vi "Curve Generator (SubVI).vi"(4 "Number of Samples":i32, 6 "Total Length (ms)":dbl, 7 "Start Amplitude (mA)":dbl, 9 "Post-ramp\nRadius (ms/mA)":dbl, 10 "Pre-ramp\nRadius (ms/mA)":dbl, 11 "End Amplitude (mA)":dbl) -> (1 "Charge (mC)":dbl, 2 "dt":dbl, 3 "S-Curve":dbl[](array[numeric]))   [LabVIEW 2020]
uses:
  <vilib>/Analysis/1siggen.llb/Ramp Pattern by Samples.vi
  <vilib>/Analysis/NI_AALBase.lvlib
panel:
  out "output variable":dbl
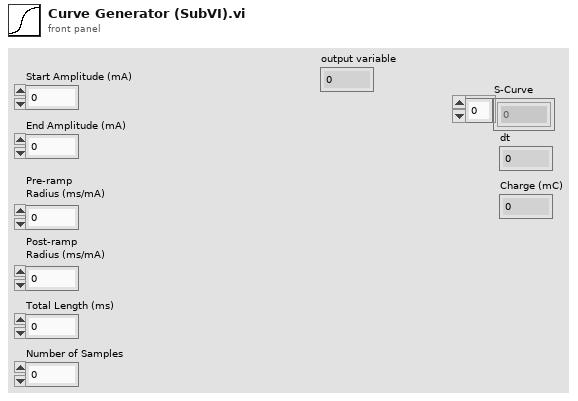
[diagram p1: front panel]
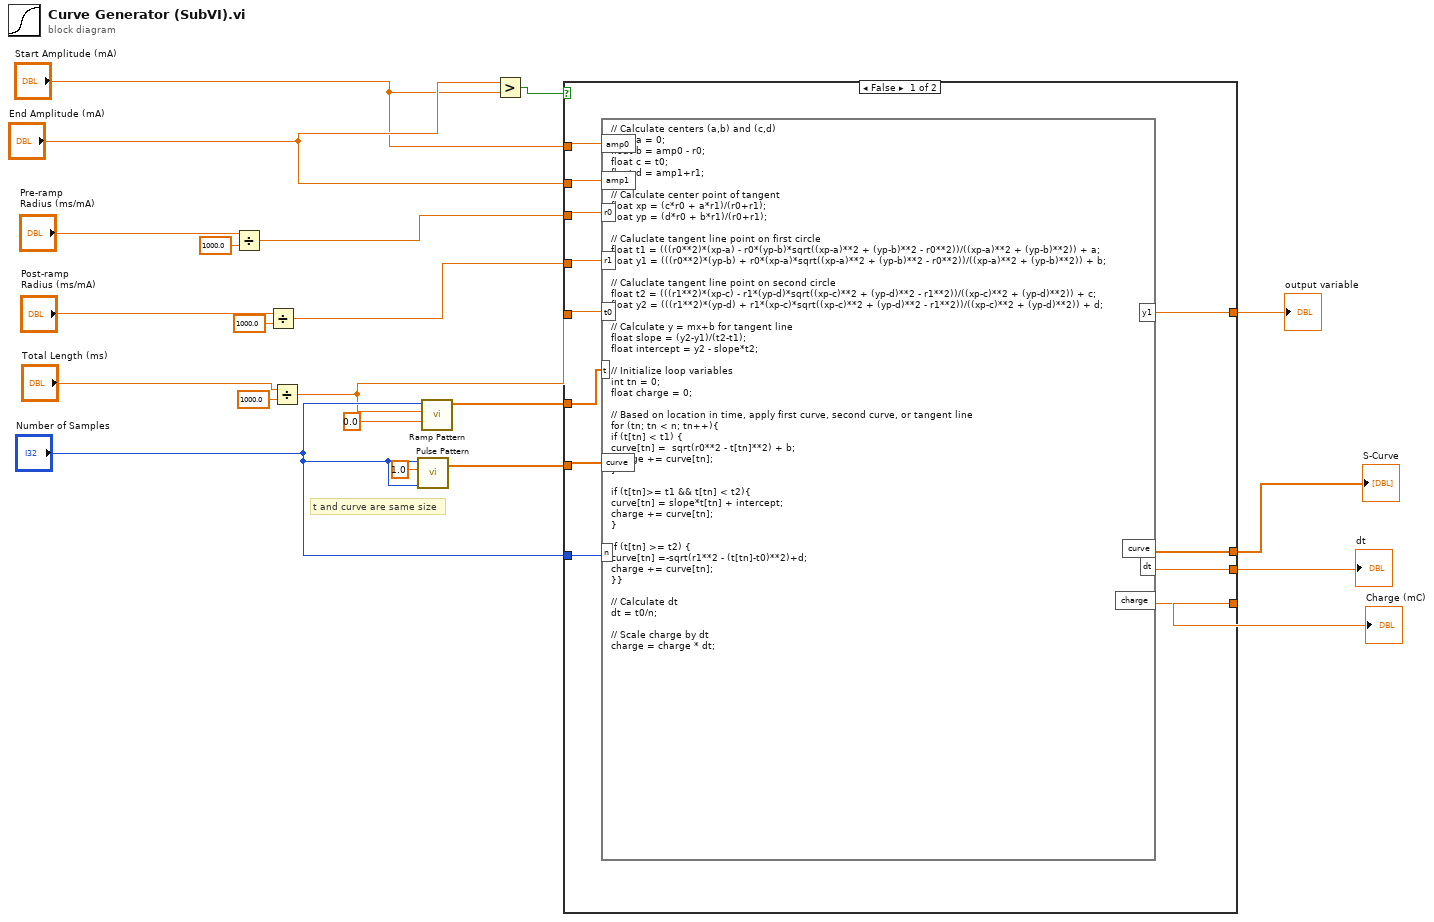
[diagram p0: block diagram]
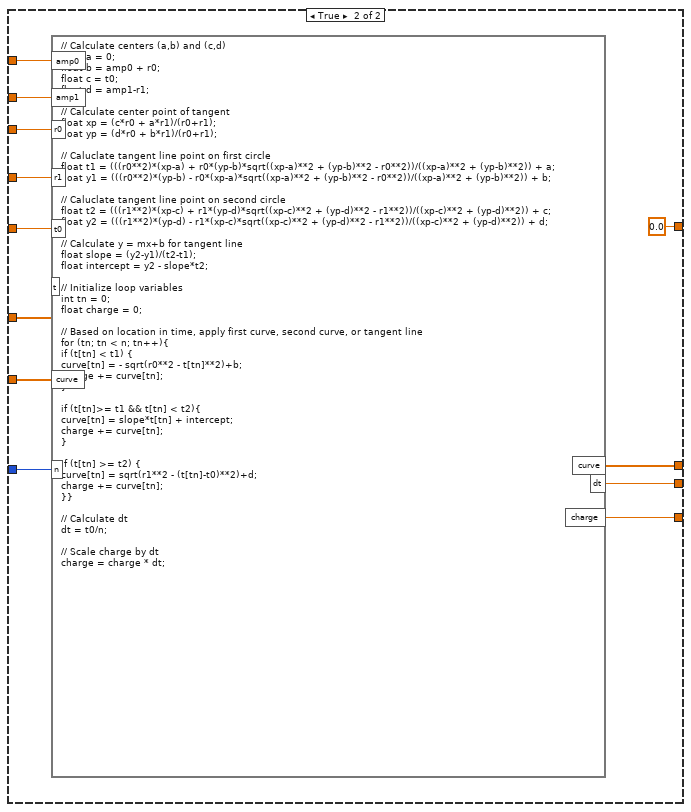
[diagram p2: hidden frame]
diagram:
  # "t and curve are same size"
  n1 = Divide(x="Pre-ramp\nRadius (ms/mA)", y=1000.0) -> (x/y=w14:dbl)
  n2 = Divide(x="Post-ramp\nRadius (ms/mA)", y=1000.0) -> (x/y=w9:dbl)
  n3 = Divide(x="Total Length (ms)", y=1000.0) -> (x/y=w10:dbl)
  n4 = call <vilib>:"Pulse Pattern.vi"("width"="Number of Samples", "amplitude"=1.0, "samples"="Number of Samples") -> ("Pulse Pattern"=w20:dbl[])  [unwired: 1 in, 1 out]
  n5 = call-poly <vilib>:"Ramp Pattern.vi"("start"=0.0, "end"=w10, "samples"="Number of Samples") -> ("Ramp Pattern"=w18:dbl[])  [unwired: 7 in, 1 out]
  n6 = Greater?(x="End Amplitude (mA)", y="Start Amplitude (mA)") -> (0:w2:bool)
  n7 = case shown="False" w2 {
    tunnel: "End Amplitude (mA)" -> [w29 w45]
    tunnel: "Number of Samples" -> [w23 w44]
    tunnel: w20 -> [w24 w43]
    tunnel: [w31 w42] -> w19
    tunnel: w18 -> [w25 w41]
    tunnel: [w32 w40] -> w17
    tunnel: "Start Amplitude (mA)" -> [w30 w39]
    tunnel: w14 -> [w28 w38]
    tunnel: w10 -> [w26 w37]
    tunnel: w9 -> [w27 w36]
    tunnel: [w33 w35] -> w7
    tunnel: [w22 0.0] -> w1
    frame False {
      n8 = formula code="// Calculate centers (a,b) and (c,d)\nfloat a = 0;\nfloat b = amp0 - r0;\nfloat c = t0;\nfloat d = amp1+r1;\n\n// Calculate center point of tangent\nfloat xp = (c*r0 + a*r1)/(r0+r1);\nfloat yp = (d*r0 + b*r1)/(r0+r1);\n\n// Caluclate tangent line point on first circle\nfloat t1 = (((r0**2)*(xp-a) - r0*(yp-b)*sqrt((xp-a)**2 + (yp-b)**2 - r0**2))/((xp-a)**2 + (yp-b)**2)) + a;\nfloat y1 = (((r0**2)*(yp-b) + r0*(xp-a)*sqrt((xp-a)**2 + (yp-b)**2 - r0**2))/((xp-a)**2 + (yp-b)**2)) + b;\n\n// Caluclate tangent line point on second circle\nfloat t2 = (((r1**2)*(xp-c) - r1*(yp-d)*sqrt((xp-c)**2 + (yp-d)**2 - r1**2))/((xp-c)**2 + (yp-d)**2)) + c;\nfloat y2 = (((r1**2)*(yp-d) + r1*(xp-c)*sqrt((xp-c)**2 + (yp-d)**2 - r1**2))/((xp-c)**2 + (yp-d)**2)) + d;\n\n// Calculate y = mx+b for tangent line\nfloat slope = (y2-y1)/(t2-t1);\nfloat intercept = y2 - slope*t2;\n\n// Initialize loop variables\nint tn = 0;\nfloat charge = 0;\n\n// Based on location in time, apply first curve, second curve, or tangent line\nfor (tn; tn < n; tn++){\nif (t[tn] < t1) {\ncurve[tn] =  sqrt(r0**2 - t[tn]**2) + b;\ncharge += curve[tn];\n}\n\nif (t[tn]>= t1 && t[tn] < t2){\ncurve[tn] = slope*t[tn] + intercept;\ncharge += curve[tn];\n}\n\nif (t[tn] >= t2) {\ncurve[tn] =-sqrt(r1**2 - (t[tn]-t0)**2)+d;\ncharge += curve[tn];\n}}\n\n// Calculate dt\ndt = t0/n;\n\n// Scale charge by dt\ncharge = charge * dt;"("amp0"=w30, "r0"=w28, "r1"=w27, "t0"=w26, "t"=w25, "n"=w23, "curve"=w24, "amp1"=w29) -> ("curve"=w33:dbl[], "dt"=w32:dbl, "charge"=w31:dbl, "y1"=w22:dbl)
    }
    frame True {
      n9 = formula code="// Calculate centers (a,b) and (c,d)\nfloat a = 0;\nfloat b = amp0 + r0;\nfloat c = t0;\nfloat d = amp1-r1;\n\n// Calculate center point of tangent\nfloat xp = (c*r0 + a*r1)/(r0+r1);\nfloat yp = (d*r0 + b*r1)/(r0+r1);\n\n// Caluclate tangent line point on first circle\nfloat t1 = (((r0**2)*(xp-a) + r0*(yp-b)*sqrt((xp-a)**2 + (yp-b)**2 - r0**2))/((xp-a)**2 + (yp-b)**2)) + a;\nfloat y1 = (((r0**2)*(yp-b) - r0*(xp-a)*sqrt((xp-a)**2 + (yp-b)**2 - r0**2))/((xp-a)**2 + (yp-b)**2)) + b;\n\n// Caluclate tangent line point on second circle\nfloat t2 = (((r1**2)*(xp-c) + r1*(yp-d)*sqrt((xp-c)**2 + (yp-d)**2 - r1**2))/((xp-c)**2 + (yp-d)**2)) + c;\nfloat y2 = (((r1**2)*(yp-d) - r1*(xp-c)*sqrt((xp-c)**2 + (yp-d)**2 - r1**2))/((xp-c)**2 + (yp-d)**2)) + d;\n\n// Calculate y = mx+b for tangent line\nfloat slope = (y2-y1)/(t2-t1);\nfloat intercept = y2 - slope*t2;\n\n// Initialize loop variables\nint tn = 0;\nfloat charge = 0;\n\n// Based on location in time, apply first curve, second curve, or tangent line\nfor (tn; tn < n; tn++){\nif (t[tn] < t1) {\ncurve[tn] = - sqrt(r0**2 - t[tn]**2)+b;\ncharge += curve[tn];\n}\n\nif (t[tn]>= t1 && t[tn] < t2){\ncurve[tn] = slope*t[tn] + intercept;\ncharge += curve[tn];\n}\n\nif (t[tn] >= t2) {\ncurve[tn] = sqrt(r1**2 - (t[tn]-t0)**2)+d;\ncharge += curve[tn];\n}}\n\n// Calculate dt\ndt = t0/n;\n\n// Scale charge by dt\ncharge = charge * dt;"("amp0"=w39, "r0"=w38, "r1"=w36, "t0"=w37, "t"=w41, "n"=w44, "curve"=w43, "amp1"=w45) -> ("curve"=w35:dbl[], "dt"=w40:dbl, "charge"=w42:dbl)
    }
  }
  "S-Curve" <- w7
  "Charge (mC)" <- w19
  "dt" <- w17
  "output variable" <- w1
